vi "Switch.vi"(2 "Input":dbl, 3 "Switch":bool) -> (0 "Output 2":dbl, 1 "Output 1":dbl)   [LabVIEW 2017]
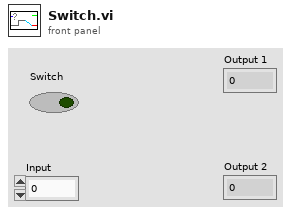
[diagram p1: front panel]
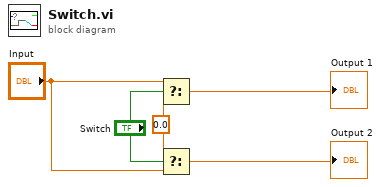
[diagram p0: block diagram]
diagram:
  w3 = 0.0 ("t")
  n1 = Select(t="Input", s="Switch", f=w3) -> (s? t:f=→"Output 1":dbl)
  n2 = Select(t=w3, s="Switch", f="Input") -> (s? t:f=→"Output 2":dbl)
